vi "ReplaceClassNameInDescription.vi"(1 "replace type descr":u8[](array[numeric]) format="%x", 3 "org class type descr":u8[](array[numeric]) format="%x") -> (15 "class type decr out":u8[](array[numeric]) format="%x")   [LabVIEW 2020, in "G#DebugServer.lvclass"]
uses:
  <vilib>/addons/_AddQ/G#DebugServer/G#DebugServer.lvclass
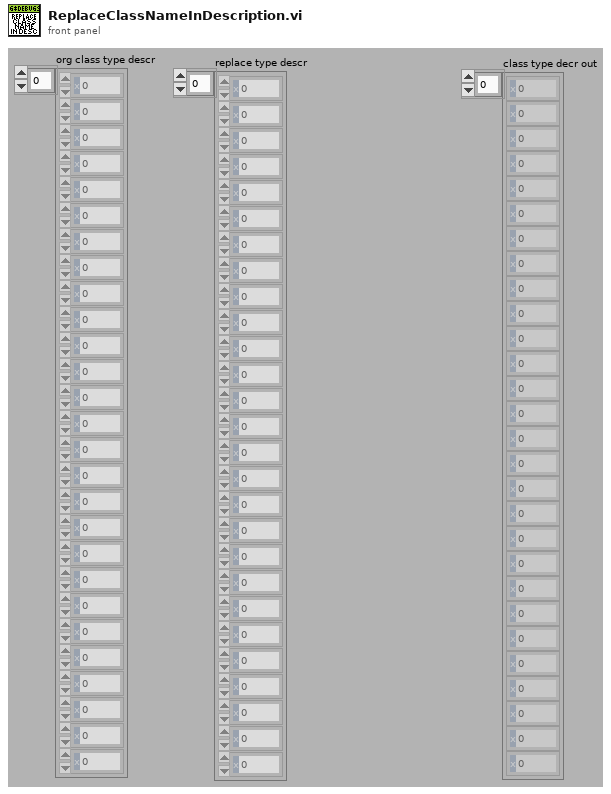
[diagram p1: front panel]
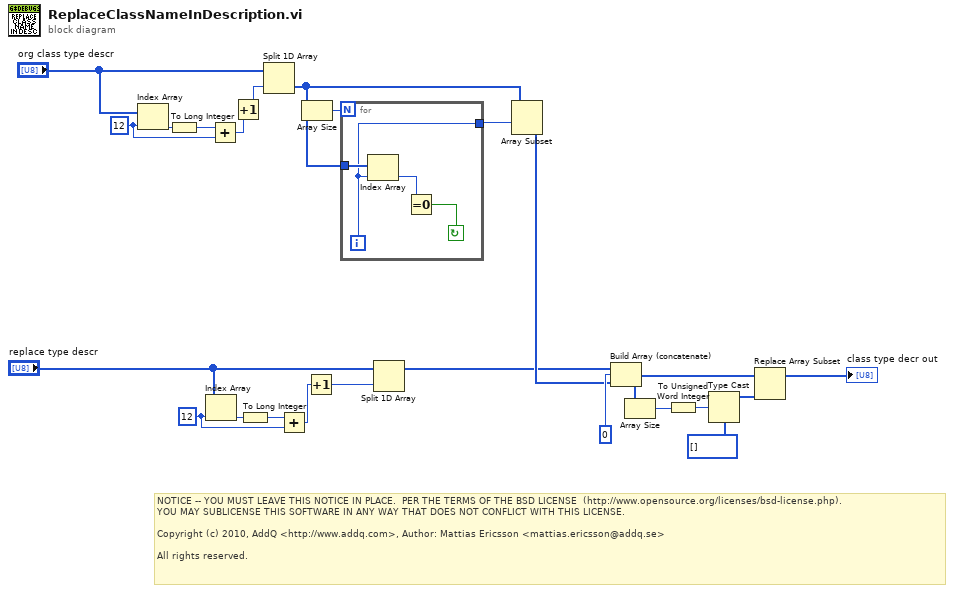
[diagram p0: block diagram]
diagram:
  w20 = 12 ("index")
  w23 = 12 ("index")
  # "NOTICE -- YOU MUST LEAVE THIS NOTICE IN PLACE.  PER THE TERMS OF THE BSD LICENSE  (http://www.opensource.org/licenses/bsd-license.php).\nYOU MAY SUBLICENSE THIS SOFTWARE IN ANY WAY THAT DOES NOT CONFLICT WITH THIS LICENSE.\n\nCopyright (c) 2010, AddQ <http://www.addq.com>, Author: Mattias Ericsson <mattias.ericsson@addq.se>\n\nAll rights reserved."
  n1 = Index Array(array="org class type descr", index=w23) -> (element=w24:u8)
  n2 = To Long Integer(number=w24) -> (32bit integer=w5:i32)
  n3 = Index Array(array="replace type descr", index=w20) -> (element=w19:u8)
  n4 = Add(x=w5, y=w23) -> (x+y=w10:i32)
  n5 = Increment(x=w10) -> (x+1=w8:i32)
  n6 = To Long Integer(number=w19) -> (32bit integer=w17:i32)
  n7 = Split 1D Array(array="org class type descr", index=w8) -> (second subarray=w9:u8[])  [unwired: 1 out]
  n8 = Add(x=w17, y=w20) -> (x+y=w18:i32)
  n9 = Array Size(array=w9) -> (size(s)=w22:i32)
  n10 = Increment(x=w18) -> (x+1=w11:i32)
  n11 = for {
    N: w22 -> [_]
    tunnel: w9 -> [w28]
    tunnel: [w25] -> w21
    i -> [w25]
    stop <- w26 continue-if-true
    n12 = Index Array(array=w28, index=w25) -> (element=w27:u8)
    n13 = Equal To 0?(x=w27) -> (x = 0?=w26:bool)
  }
  n14 = Split 1D Array(array="replace type descr", index=w11) -> (first subarray=w3:u8[])  [unwired: 1 out]
  n15 = Array Subset(array=w9, index=w21) -> (w6:u8[])  [unwired: 1 in]
  n16 = Build Array (concatenate)(w3, u8 0, w6) -> (w13:u8[])
  n17 = Array Size(array=w13) -> (size(s)=w15:i32)
  n18 = To Unsigned Word Integer(number=w15) -> (unsigned 16bit integer=w12:u16)
  n19 = Type Cast(type=u8[] [] ("ReplaceTypeDesct"), x=w12) -> (*(type *) &x=w14:u8[])
  n20 = Replace Array Subset(array=w13, new element=w14) -> (→"class type decr out":u8[])  [unwired: 1 in]
